vi "Normalized_Mutual_Info_Score.vi"(8 "error in (no error)":errorcluster caption="entrée d'erreur (pas d'erreur)", 9 "labels_pred":string[][](array[string]), 10 "labels_true":string[][](array[string]), 11 "normalized_mutual_info_score":cluster{"average_method":string}={"average_method"="arithmetic"}) -> (0 "error out":errorcluster caption="sortie d'erreur", 3 "Score":string)   [LabVIEW 2020]
doc: "Normalized Mutual Information between two clusterings.\n\nNormalized Mutual Information (NMI) is a normalization of the Mutual Information (MI) score to scale the results between 0 (no mutual information) and 1 (perfect correlation). In this function, mutual information is normalized by some generalized mean of H(labels_true) and H(labels_pred)), defined by the average_method.\n\nThis measure is not adjusted for chance. Therefore adjusted_mutual_info_score might be preferred.\n\nThis metric is independent of the absolute values of the labels: a permutation of the class or cluster label values won’t change the score value in any way.\n\nThis metric is furthermore symmetric: switching label_true with label_pred will return the same score value. This can be useful to measure the agreement of two independent label assignments strategies on the same dataset when the real ground truth is not known.\n\n\n\n\nParameters : \n\n- labels_true : int array, shape = [n_samples]\nA clustering of the data into disjoint subsets.\n\n- labels_pred : int array-like of shape (n_samples,)\nA clustering of the data into disjoint subsets.\n\n- average_method : string, optional (default: ‘arithmetic’)\nHow to compute the normalizer in the denominator. Possible options are ‘min’, ‘geometric’, ‘arithmetic’, and ‘max’.\n\nReturns :\n\n- nmi : float\nscore between 0.0 and 1.0. 1.0 stands for perfectly complete labeling"
uses:
  Normalized_Mutual_Info_Score.lvclass
panel:
  out "Normalized_Mutual_Info_Score.lvclass":refnum<class "Normalized_Mutual_Info_Score.lvclass">
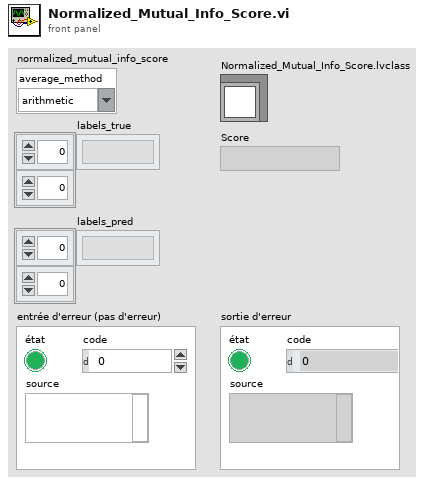
[diagram p1: front panel]
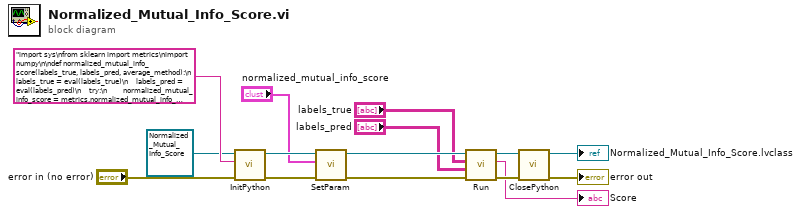
[diagram p0: block diagram]
diagram:
  n1 = call-dynamic "InitPython.vi"("error in (no error)"="error in (no error)", "Python Instruction"="import sys\nfrom sklearn import metrics\nimport numpy\n\ndef normalized_mutual_info_score(labels_true, labels_pred, average_method):\n    labels_true = eval(labels_true)\n    labels_pred = eval(labels_pred)\n    try:\n        normalized_mutual_info_score = metrics.normalized_mutual_info_score(labels_true, labels_pred, average_method)\n        normalized_mutual_info_score = normalized_mutual_info_score.tolist()\n        return str(normalized_mutual_info_score)\n    except:\n        erreur = sys.exc_info()\n        typerr = u\"%s\" % (erreur[0])\n        typerr = typerr[typerr.find(\"'\")+1:typerr.rfind(\"'\")]\n        msgerr = u\"%s\" % (erreur[1])\n        message = str('/!\\\\ {0} : {1}'. format(typerr,msgerr))\n        return message", "Scikit-learn en entrée"=refnum<class "Normalized_Mutual_Info_Score.lvclass"> refnum ("Normalized_Mutual_Info_Score.lvclass")) -> ("error out"=w9:errorcluster, "Scikit-learn en sortie"=w11:refnum<class "Normalized_Mutual_Info_Score.lvclass">)  [unwired: 7 in]
  n2 = call-dynamic "SetParam.vi"("error in (no error)"=w9, "normalized_mutual_info_score"="normalized_mutual_info_score", "Normalized_Mutual_Info_Score.lvclass"=w11) -> ("error out"=w7:errorcluster, "Normalized_Mutual_Info_Score.lvclass"=w8:refnum<class "Normalized_Mutual_Info_Score.lvclass">)  [unwired: 7 in]
  n3 = call-dynamic "Run.vi"("error in (no error)"=w7, "labels_pred"="labels_pred", "labels_true"="labels_true", "Normalized_Mutual_Info_Score.lvclass"=w8) -> ("error out"=w5:errorcluster, "String Data"=→"Score":string, "Normalized_Mutual_Info_Score.lvclass"=w6:refnum<class "Normalized_Mutual_Info_Score.lvclass">)  [unwired: 5 in]
  n4 = call-dynamic "ClosePython.vi"("error in (no error)"=w5, "Scikit-learn en entrée"=w6) -> ("error out"=→"error out":errorcluster, "Scikit-learn en sortie"=→"Normalized_Mutual_Info_Score.lvclass":refnum<class "Normalized_Mutual_Info_Score.lvclass">)  [unwired: 8 in]
